vi "TRANSFER ITEMS.vi"(10 "REFERENCES":T3, 11 "DATA IN":T2[](array[typedef])) -> (2 "USER/ITEM DATA TRANSFER OUT":T1(array[cluster]), 3 "DATA OUT":T2[](array[typedef]))   [LabVIEW 2019]
uses:
  Controls/References Cluster.ctl
  <vilib>/userDefined/High Color/IMAQdx.ctl
  Controls/Custom Calendar/Custom Calendar.xctl
  Controls/Table Data Types/Inventory Data Type.ctl
  Controls/Table Data Types/User Data Type.ctl
  Controls/Column Names/Inventory Column Names.ctl
  <vilib>/addons/database/Connection.llb/DB Tools Open Connec (String).vi
  <vilib>/addons/database/Connection.llb/Conn Execute.vi
  <vilib>/addons/database/Recordset.llb/Rec Fetch Recordset Data (R).vi
  <vilib>/addons/database/Recordset.llb/Rec Destroy - Connection.vi
  <vilib>/addons/database/_DB Variant To Data/Database Variant To Data.xnode
  <vilib>/addons/database/NI_Database_API.lvlib
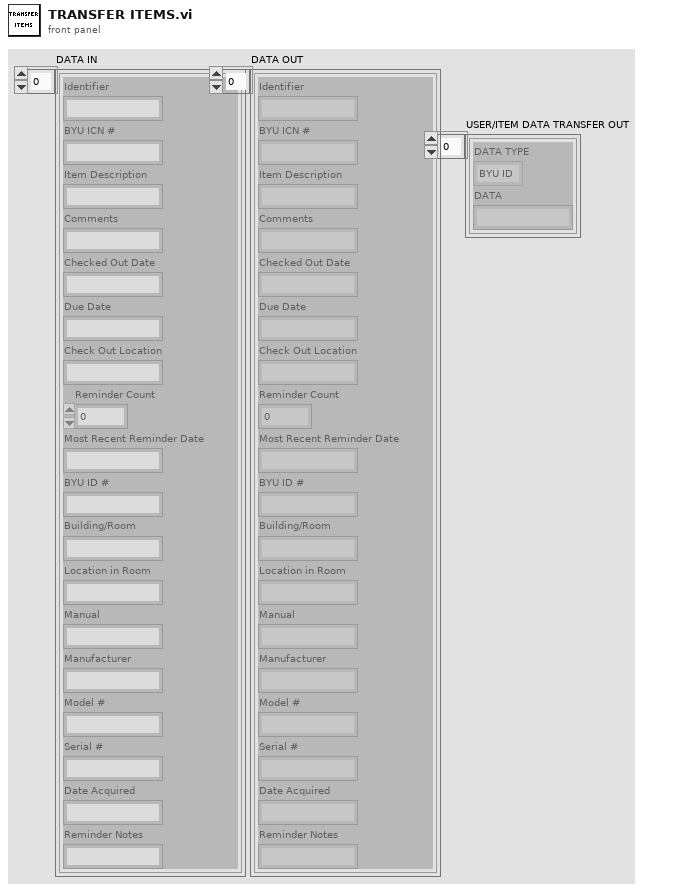
[diagram p1: front panel]
types:
  T1 = cluster{"DATA TYPE":enum16{"BYU ID", "ME#/IDENTIFIER", "BYU ICN"}, "DATA":string}[]
  T2 = typedef "Inventory Data Type.ctl" = cluster{"Identifier":string, "BYU ICN #":string, "Item Description":string, "Comments":string, "Checked Out Date":string, "Due Date":string, "Check Out Location":string, "Reminder Count":i32, "Most Recent Reminder Date":string, "BYU ID #":string, "Building/Room":string, "Location in Room":string, "Manual":string, "Manufacturer":string, "Model #":string, "Serial #":string, "Date Acquired":string, "Reminder Notes":string}
  T3 = typedef "References Cluster.ctl" = cluster{"MAIN PAGES":refnum<vi>, "ADD/EDIT ITEM REFERENCES":cluster{"Identifier":refnum<vi>, "BYU ICN #":refnum<vi>, "Item Description":refnum<vi>, "Comments":refnum<vi>, "Checked Out Date":refnum<vi>, "Due Date":refnum<vi>, "Check Out Location":refnum<vi>, "Reminder Count":refnum<vi>, "Most Recent Reminder Date":refnum<vi>, "BYU ID #":refnum<vi>, "Building/Room":refnum<vi>, "Location in Room":refnum<vi>, "Manual":refnum<vi>, "Manufacturer":refnum<vi>, "Model #":refnum<vi>, "Serial #":refnum<vi>, "Date Acquired":refnum<vi>, "ADD/EDIT ITEM LABEL":refnum<vi>, "ARCHIVE ITEM":refnum<vi>, "Archive Item Inputs":refnum<vi>, "Reminder Notes":refnum<vi>, "DUPLICATE ITEM":refnum<vi>}, "ADD/EDIT USER REFERENCES":cluster{"BYU ID # (##-###-####)":refnum<vi>, "First Name":refnum<vi>, "Last Name":refnum<vi>, "Phone Number (###-###-####)":refnum<vi>, "Email":refnum<vi>, "Department":refnum<vi>, "Graduation Status":refnum<vi>, "Anticipated Graduation Year":refnum<vi>, "Credit Score":refnum<vi>, "Date Added":refnum<vi>, "Graduation Clearance Date":refnum<vi>, "Picture File Name":refnum<vi>, "ADD/EDIT USER LABEL":refnum<vi>, "Department Map":refnum<vi>, "Status Map":refnum<vi>, "Anticipated Graduation Year Map":refnum<vi>, "User Agreement":refnum<vi>, "User Comments":refnum<vi>, "Camera":refnum<vi>}, "RETURN ITEM REFERENCES":cluster{"Item or Person:":refnum<vi>, "Search Return Results":refnum<vi>, "What are you searching for?":refnum<vi>}, "SEARCH DATABASE REFERENCES":cluster{"What to Search For:":refnum<vi>, "Where to Search":refnum<vi>, "Column to Search In":refnum<vi>, "Column to Sort By":refnum<vi>, "Search Database Results":refnum<vi>, "Inventory Column Selector":refnum<vi>, "User Column Selector":refnum<vi>, "Inventory Archive Column Selector":refnum<vi>, "User Archive Column Selector":refnum<vi>, "Sales Tracking Column Selector":refnum<vi>, "Checked In Archive Column Selector":refnum<vi>, "Restore User":refnum<vi>, "Date Range":refnum<vi>, "Dates Less Than":refnum<vi>, "Dates Greater Than":refnum<vi>, "Search Print Receipt":refnum<vi>, "Edit Sale Description":refnum<vi>}, "USER ITEMS REFERENCES":cluster{"USER'S INFORMATION":refnum<vi>, "User's Checked Out Items":refnum<vi>, "User Info Comments":refnum<vi>, "SEE USER INFO COMMENTS":refnum<vi>}, "EDIT ITEMS REFERENCES":cluster{"New Check Out Location":refnum<vi>, "Items to Edit":refnum<vi>, "Edit Items Due Date":refnum<vi>, "New Reminder Notes":refnum<vi>, "New Item Description":refnum<vi>}, "CHECK OUT ITEMS REFERENCES":cluster{"Enter Item:":refnum<vi>, "Check Out Items Due Date":refnum<vi>, "Check Out Location":refnum<vi>, "Items to be Checked Out":refnum<vi>, "Possible Items":refnum<vi>, "Altered Item Description":refnum<vi>}, "TRANSFER ITEMS REFERENCES":cluster{"Search Parameter":refnum<vi>, "What to Match":refnum<vi>, "Matching Individuals":refnum<vi>, "Items to be Transferred":refnum<vi>}, "SETTINGS REFERENCES":cluster{"PSC Database Settings":refnum<vi>, "PSC Sales Item Spreadsheet":refnum<vi>}, "PSC SALES REFERENCES":cluster{"BYU ID CARD #":refnum<vi>, "Sale Description":refnum<vi>, "Scan or Enter Item Name":refnum<vi>, "Items to be Sold":refnum<vi>, "Grand Total":refnum<vi>, "Item List":refnum<vi>}}
  T4 = cluster{"DATA TYPE":enum16{"BYU ID", "ME#/IDENTIFIER", "BYU ICN"}, "DATA":string}
  T5 = typedef "User Data Type.ctl" = cluster{"BYU ID #":string, "First Name":string, "Last Name":string, "Phone Number":string, "Email":string, "Department":string, "Graduation Status":string, "Anticipated Graduation Year":string, "Credit Score":dbl, "Date Added":string, "Graduation Clearance Date":string, "Picture File Name":string, "User Comments":string}
  T6 = cluster{"Search Parameter":refnum<vi>, "What to Match":refnum<vi>, "Matching Individuals":refnum<vi>, "Items to be Transferred":refnum<vi>}
  T7 = typedef "NI_Database_API.lvlib/Conn ObjectReference.ctl" = refnum<k1>
  T8 = typedef "NI_Database_API.lvlib/Rec ObjectReference.ctl" = refnum<k1>
  T9 = typedef "Inventory Column Names.ctl" = string[]
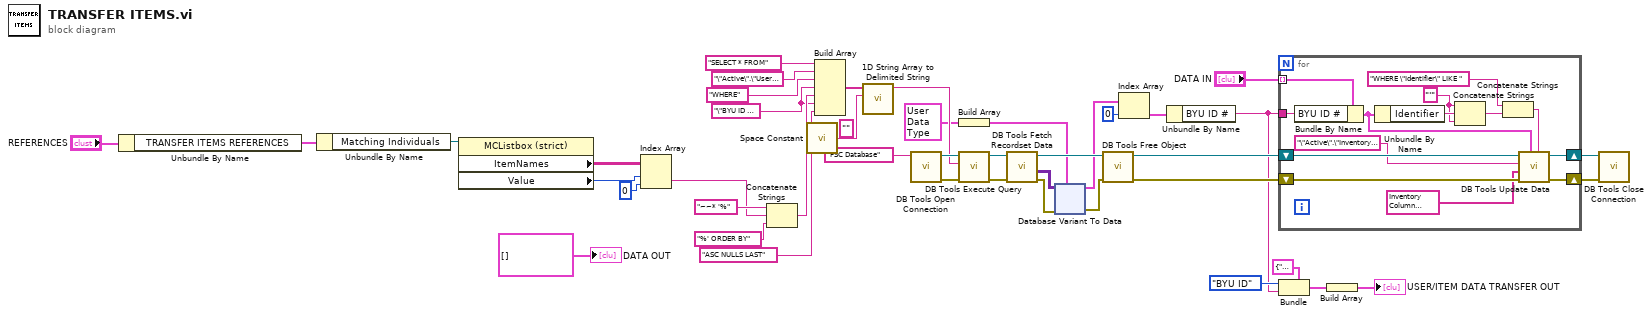
[diagram p0: block diagram]
diagram:
  w5 = "\"BYU ID #\"" ("element")
  (unwired) "" ("element")
  n1 = Unbundle By Name("REFERENCES") -> ("TRANSFER ITEMS REFERENCES"=w42:T6)
  n2 = Unbundle By Name(w42) -> ("Matching Individuals"=w6:refnum<vi>)
  n3 = property class="MCListbox (strict)"(reference=w6) -> ("ItemNames"=w4:string[][], "Value"=w3:i32)  [unwired: 1 in, 2 out]
  n4 = Index Array(array=w4, index (row)=w3, index (col)=0 ("disabled index (col)")) -> (element=w1:string)
  n5 = Concatenate Strings("~~* '%", w1, "%' ORDER BY") -> (w33:string)
  n6 = call <vilib>:"Space Constant.vi"() -> ("String"=w30:string)
  n7 = Build Array("SELECT * FROM", "\"Active\".\"Users\"", "WHERE", w5, w33, w5, "ASC NULLS LAST") -> (w31:string[])
  n8 = call <vilib>:"1D String Array to Delimited String.vi"("delimiter"=w30, "string array"=w31) -> ("delimited string"=w29:string)  [unwired: 9 in]
  n9 = call-poly <vilib>:"DB Tools Open Connection.vi"("connection information"="PSC Database") -> ("error out"=w39:errorcluster, "connection reference"=w40:T7)  [unwired: 7 in]
  n10 = Build Array(T5 {"BYU ID #"="", "First Name"="", "Last Name"="", "Phone Number"="", "Email"="", "Department"="", "Graduation Status"="", "Anticipated Graduation Year"="", "Credit Score"=0.0, "Date Added"="", "Graduation Clearance Date"="", "Picture File Name"="", "User Comments"=""} ("Array")) -> (w7:T5[])
  n11 = call-poly <vilib>:"DB Tools Execute Query.vi"("error in (no error)"=w39, "SQL query"=w29, "connection reference"=w40) -> ("error out"=w27:errorcluster, "recordset reference"=w28:T8)  [unwired: 5 in]
  n12 = call-poly <vilib>:"DB Tools Fetch Recordset Data.vi"("error in (no error)"=w27, "recordset reference"=w28) -> ("error out"=w25:errorcluster, "recordset data"=w26:variant[][], "recordset reference out"=w24:T8)  [unwired: 3 in]
  n13 = xnode "Database Variant To Data"("database variant"=w26, "error in (no error)"=w25, "type"=w7) -> ("data"=w22:T5[], "error out"=w23:errorcluster)
  n14 = call-poly <vilib>:"DB Tools Free Object.vi"("error in (no error)"=w23, "recordset reference"=w24) -> ("error out"=w16:errorcluster, "connection reference"=w17:T7)  [unwired: 8 in]
  n15 = Index Array(array=w22, index=0) -> (element=w19:T5)
  n16 = Unbundle By Name(w19) -> ("BYU ID #"=w13:string)
  n17 = for {
    tunnel: w13 -> [w56]
    tunnel: "DATA IN" -> [w57] mode=indexing
    shift-right: [w49] -> w9
    shift-left: w16 -> [w51]
    shift-right: [w50] -> w10
    shift-left: w17 -> [w52]
    w45 = "'"
    n18 = Bundle By Name(cluster=w57, "BYU ID #"=w56) -> (w54:T2)
    n19 = Unbundle By Name(w54) -> ("Identifier"=w46:string)
    n20 = Concatenate Strings(w45, w46, w45) -> (w47:string)
    n21 = Concatenate Strings("WHERE \"Identifier\" LIKE ", w47) -> (w53:string)
    n22 = call <vilib>:"DB Tools Update Data.vi"("condition"=w53, "data"=w54, "error in (no error)"=w51, "columns"=T9 ["\"Identifier\"", "\"BYU ICN #\"", "\"Item Description\"", "\"Comments\"", "\"Checked Out Date\"", "\"Due Date\"", "\"Check Out Location\"", "\"Reminder Count\"", "\"Most Recent Reminder Date\"", "\"BYU ID #\"", "\"Building/Room\"", "\"Location in Room\"", "\"Manual\"", "\"Manufacturer\"", "\"Model #\"", "\"Serial #\"", "\"Date Acquired\"", "\"Reminder Notes\""] ("INVENTORY COLUMN NAMES"), "table"="\"Active\".\"Inventory\"", "connection reference"=w52) -> ("error out"=w49:errorcluster, "connection reference out"=w50:T7)  [unwired: 4 in]
  }
  n23 = Bundle(cluster=T4 {"DATA TYPE"=enum."BYU ID", "DATA"=""} ("USER/ITEM DATA TRANSFER"), "DATA TYPE"=enum16{"BYU ID", "ME#/IDENTIFIER", "BYU ICN"}."BYU ID", "DATA"=w13) -> (w12:T4)
  n24 = Build Array(w12) -> (→"USER/ITEM DATA TRANSFER OUT":T1)
  n25 = call <vilib>:"DB Tools Close Connection.vi"("error in (no error)"=w9, "connection reference"=w10) -> ()  [unwired: 5 in, 1 out]
  "DATA OUT" <- T2[] [] ("DATA OUT")
